vi "2D数组排序[CSG 实部,虚部](冲突时的文件备份2013-05-03 10-41-21).vi"(7 "升降序":enum16{"升序", "降序"}(ring), 8 "error in (no error)":errorcluster caption="错误输入（无错误）", 9 "选择行列":enum16{"行", "列"}(ring), 10 "行/列索引":i32, 11 "输入数组":csg[][](array[numeric])) -> (0 "error out":errorcluster caption="错误输出", 2 "排序后索引":i32[](array[numeric]), 3 "排序后数组":csg[][](array[numeric]) format="%.2f")   [LabVIEW 2012]
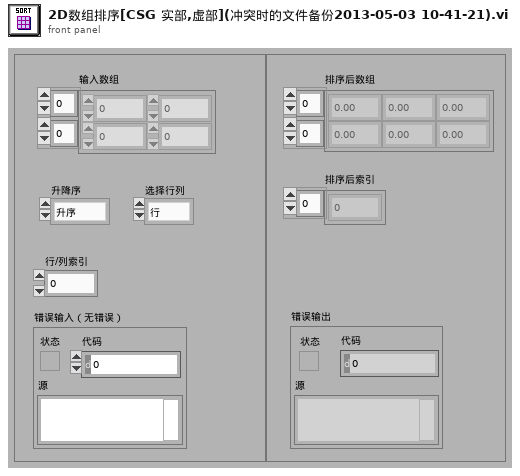
[diagram p1: front panel]
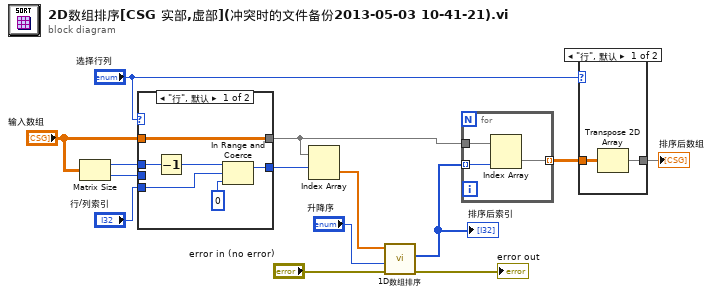
[diagram p0: block diagram]
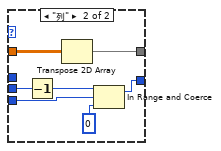
[diagram p3: hidden frame]
diagram:
  n1 = Matrix Size(0:"输入数组") -> (1:w14:i32, 2:w13:i32)
  n2 = case shown="\"行\", 默认" "选择行列" {
    tunnel: w14 -> [w20 _]
    tunnel: w13 -> [_ w26]
    tunnel: "行/列索引" -> [w16 w21]
    tunnel: [w18 w25] -> w7
    tunnel: "输入数组" -> [w17 w24]
    tunnel: [w17 w23] -> w4
    frame "行", Default {
      n3 = Decrement(x=w20) -> (x-1=w15:i32)
      n4 = In Range and Coerce(upper limit=w15, x=w16, lower limit=0 ("下限")) -> (coerced(x)=w18:i32)  [unwired: 1 out]
    }
    frame "列" {
      n5 = Decrement(x=w26) -> (x-1=w22:i32)
      n6 = Transpose 2D Array(2D array=w24) -> (transposed array=w23:csg[][])
      n7 = In Range and Coerce(upper limit=w22, x=w21, lower limit=0 ("下限")) -> (coerced(x)=w25:i32)  [unwired: 1 out]
    }
  }
  n8 = Index Array(array=w4, index (row)=w7) -> (element=w10:csg[])  [unwired: 1 in]
  n9 = call-poly "1D数组排序.vi"("error in (no error)"="error in (no error)", "升降序"="升降序", "输入数组"=w10) -> ("error out"=→"error out":errorcluster, "排序后索引"=w3:i32[])  [unwired: 6 in, 1 out]
  "排序后索引" <- w3
  n10 = for {
    tunnel: w4 -> [w30]
    tunnel: w3 -> [w29] mode=indexing
    tunnel: [w28] -> w2 mode=indexing
    n11 = Index Array(array=w30, index (col)=w29) -> (element=w28:csg[])  [unwired: 1 in]
  }
  n12 = case shown="\"行\", 默认" "选择行列" {
    tunnel: [w32 w33] -> w5
    tunnel: w2 -> [w31 w33]
    frame "行", Default {
      n13 = Transpose 2D Array(2D array=w31) -> (transposed array=w32:csg[][])
    }
    frame "列" {
    }
  }
  "排序后数组" <- w5
